vi "CutWaveform.vi"(11 "SGL":waveform(sgl)[](array[waveform])) -> (3 "DBL":waveform(sgl)[](array[waveform]))   [LabVIEW 2016, in "McsaAnalysisFunctions.lvlib"]
uses:
  <vilib>/addons/InsightCM/Utilities/Analysis/MCSA/McsaAnalysisFunctions.lvlib
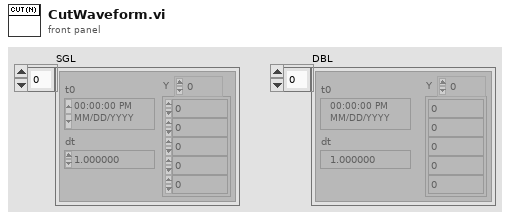
[diagram p1: front panel]
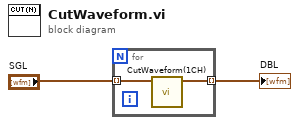
[diagram p0: block diagram]
diagram:
  n1 = for {
    tunnel: "SGL" -> [w4] mode=indexing
    tunnel: [w3] -> w1 mode=indexing
    n2 = call <vilib>:"CutWaveform(1CH).vi"("Waveform in"=w4) -> ("Waveform out"=w3:waveform(sgl))  [unwired: 10 in]
  }
  "DBL" <- w1
